vi "TEST_Check_ResistorV1.vi"(7 "ATP Check":bool, 8 ".ChA/!ChB":bool, 10 "Inputs":cluster{" Ohms":dbl, "Level OUt":dbl}={" Ohms"=101.0, "Level OUt"=7.73}) -> (1 "Level Out":T2={"Switched"=FALSE, "Level OUt"=8.494999999999996}, 2 "Err Num":i32, 3 "ChA Spec RNG Out":T3={"Specs"=[7.785, 7.685, 8.5, 202.0, 198.0, 102.0, 98.0], "LUT Status"={"ChA/!ChB"=FALSE, "Drain/!Fill"=FALSE, "In Range?"=TRUE, "Switch Range?"=FALSE, "Measure R?"=FALSE, "Vaild R?"=FALSE, "Index(n)"=2, "Index(n-1)"=1, "Index Max"=13}})   [LabVIEW 2024]
uses:
  Control Definitions/Def Spec RNG.ctl
  Control Definitions/Ded LUT_Status.ctl
  Control Definitions/Def_LevelSwitched.ctl
  Control Definitions/Def Results2.ctl
panel:
  in  "Drain/!Fill":bool
  in  "LUT Status.Index(n)":i32=2
  out "Results out":T1=[[{"Fill"=0.0, "Drain"=0.0, "Status"=0, "Resistor"=0.0}, {"Fill"=0.0, "Drain"=0.0, "Status"=0, "Resistor"=0.0}], [{"Fill"=0.0, "Drain"=0.0, "Status"=8, "Resistor"=0.0}, {"Fill"=0.0, "Drain"=0.0, "Status"=0, "Resistor"=0.0}], [{"Fill"=0.0, "Drain"=0.0, "Status"=0, "Resistor"=0.0}, {"Fill"=0.0, "Drain"=0.0, "Status"=0, "Resistor"=0.0}], [{"Fill"=0.0, "Drain"=0.0, "Status"=0, "Resistor"=0.0}, {"Fill"=0.0, "Drain"=0.0, "Status"=0, "Resistor"=0.0}], [{"Fill"=0.0, "Drain"=0.0, "Status"=0, "Resistor"=0.0}, {"Fill"=0.0, "Drain"=0.0, "Status"=0, "Resistor"=0.0}], [{"Fill"=0.0, "Drain"=0.0, "Status"=0, "Resistor"=0.0}, {"Fill"=0.0, "Drain"=0.0, "Status"=0, "Resistor"=0.0}], [{"Fill"=0.0, "Drain"=0.0, "Status"=0, "Resistor"=0.0}, {"Fill"=0.0, "Drain"=0.0, "Status"=0, "Resistor"=0.0}], [{"Fill"=0.0, "Drain"=0.0, "Status"=0, "Resistor"=0.0}, {"Fill"=0.0, "Drain"=0.0, "Status"=0, "Resistor"=0.0}], [{"Fill"=0.0, "Drain"=0.0, "Status"=0, "Resistor"=0.0}, {"Fill"=0.0, "Drain"=0.0, "Status"=0, "Resistor"=0.0}], [{"Fill"=0.0, "Drain"=0.0, "Status"=0, "Resistor"=0.0}, {"Fill"=0.0, "Drain"=0.0, "Status"=0, "Resistor"=0.0}], [{"Fill"=0.0, "Drain"=0.0, "Status"=0, "Resistor"=0.0}, {"Fill"=0.0, "Drain"=0.0, "Status"=0, "Resistor"=0.0}]] {"Resistor" format="%.1f"; "Drain" format="%.3f"; "Fill" format="%.3f"}
  in  "stop":bool
  # "ATP Check & !Valid R?\nLights Level at Index(n) -1\n\n Vaild R?\nlights Resits at Index(n-1) -1\n\n Vaild R? & Measure R?\ninserts Ohms  at Index(n-1) -1"
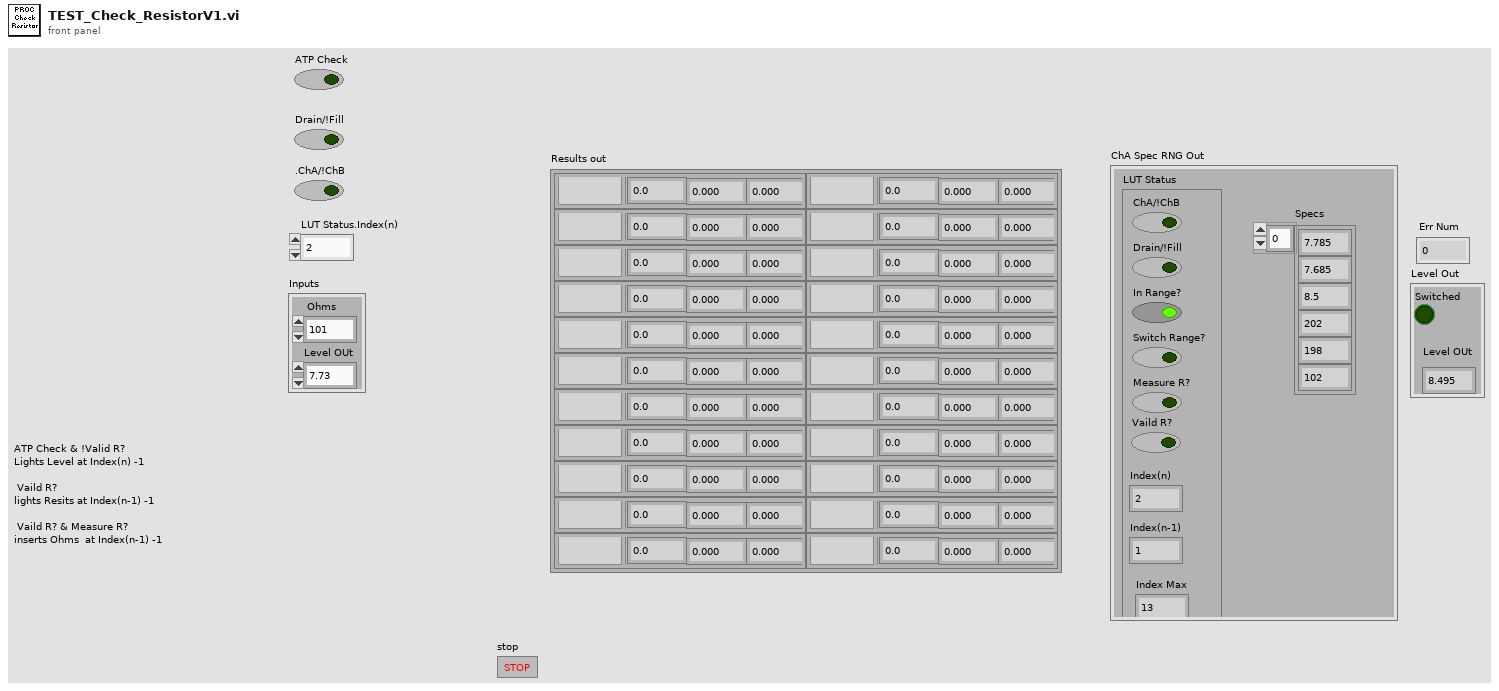
[diagram p1: front panel]
types:
  T1 = typedef "Def Results2.ctl" = cluster{"Fill":dbl, "Drain":dbl, "Status":i16, "Resistor":dbl}[][]
  T2 = typedef "Def_LevelSwitched.ctl" = cluster{"Switched":bool, "Level OUt":dbl}
  T3 = typedef "Def Spec RNG.ctl" = cluster{"Specs":dbl[], "LUT Status":T4}
  T4 = typedef "Ded LUT_Status.ctl" = cluster{"ChA/!ChB":bool, "Drain/!Fill":bool, "In Range?":bool, "Switch Range?":bool, "Measure R?":bool, "Vaild R?":bool, "Index(n)":i32, "Index(n-1)":i32, "Index Max":i32}
  T5 = cluster{"Fill":dbl, "Drain":dbl, "Status":i16, "Resistor":dbl}[]
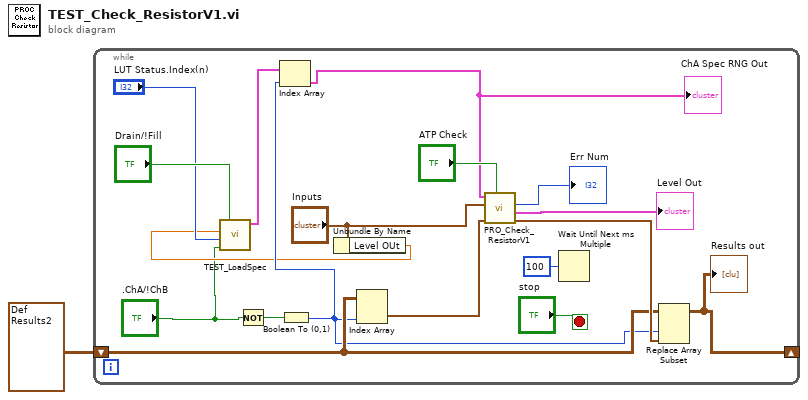
[diagram p0: block diagram]
diagram:
  n1 = while {
    shift-right: [w11] -> _
    shift-left: T1 [[{"Fill"=0.0, "Drain"=0.0, "Status"=0, "Resistor"=0.0}, {"Fill"=0.0, "Drain"=0.0, "Status"=0, "Resistor"=0.0}], [{"Fill"=0.0, "Drain"=0.0, "Status"=0, "Resistor"=0.0}, {"Fill"=0.0, "Drain"=0.0, "Status"=0, "Resistor"=0.0}], [{"Fill"=0.0, "Drain"=0.0, "Status"=0, "Resistor"=0.0}, {"Fill"=0.0, "Drain"=0.0, "Status"=0, "Resistor"=0.0}], [{"Fill"=0.0, "Drain"=0.0, "Status"=0, "Resistor"=0.0}, {"Fill"=0.0, "Drain"=0.0, "Status"=0, "Resistor"=0.0}], [{"Fill"=0.0, "Drain"=0.0, "Status"=0, "Resistor"=0.0}, {"Fill"=0.0, "Drain"=0.0, "Status"=0, "Resistor"=0.0}], [{"Fill"=0.0, "Drain"=0.0, "Status"=0, "Resistor"=0.0}, {"Fill"=0.0, "Drain"=0.0, "Status"=0, "Resistor"=0.0}], [{"Fill"=0.0, "Drain"=0.0, "Status"=0, "Resistor"=0.0}, {"Fill"=0.0, "Drain"=0.0, "Status"=0, "Resistor"=0.0}], [{"Fill"=0.0, "Drain"=0.0, "Status"=0, "Resistor"=0.0}, {"Fill"=0.0, "Drain"=0.0, "Status"=0, "Resistor"=0.0}], [{"Fill"=0.0, "Drain"=0.0, "Status"=0, "Resistor"=0.0}, {"Fill"=0.0, "Drain"=0.0, "Status"=0, "Resistor"=0.0}], [{"Fill"=0.0, "Drain"=0.0, "Status"=0, "Resistor"=0.0}, {"Fill"=0.0, "Drain"=0.0, "Status"=0, "Resistor"=0.0}], [{"Fill"=0.0, "Drain"=0.0, "Status"=0, "Resistor"=0.0}, {"Fill"=0.0, "Drain"=0.0, "Status"=0, "Resistor"=0.0}]] ("Results out") -> [w12]
    stop <- "stop" stop-if-true
    n2 = Not(x=".ChA/!ChB") -> (.not. x?=w10:bool)
    n3 = Boolean To (0,1)(Boolean=w10) -> (0, 1=w8:i16)
    n4 = Unbundle By Name("Inputs") -> ("Level OUt"=w4:dbl)
    n5 = call "TEST_LoadSpec.vi"("Drain!Fill"="Drain/!Fill", "Cha!Chb"=".ChA/!ChB", "Index"="LUT Status.Index(n)", "Level IN inches"=w4) -> ("Array"=w9:T3[])  [unwired: 6 in, 1 out]
    n6 = Index Array(array=w9, index=w8) -> (element=w2:T3)
    "ChA Spec RNG Out" <- w2
    n7 = Index Array(array=w12, index (col)=w8) -> (element=w14:T5)  [unwired: 1 in]
    n8 = call "PRO_Check_ResistorV1.vi"("ATP Check"="ATP Check", "Results IN"=w14, "Inputs"="Inputs", "ChA Spec RNG In"=w2) -> ("results out"=w13:T5, "Level Out"=→"Level Out":T2, "Err Num"=→"Err Num":i32)  [unwired: 3 in, 2 out]
    n9 = Wait Until Next ms Multiple(millisecond multiple=u32 100) -> ()  [unwired: 1 out]
    n10 = Replace Array Subset(array=w12, new element=w13, index (col)=w8) -> (w11:T1)  [unwired: 1 in]
    "Results out" <- w11
  }
